vi "Amplifier.vi"(8 "error in (no error)":errorcluster, 10 "Waveform in":waveform(dbl), 11 "RFID system in":refnum<class "RFID system.lvclass">) -> (0 "error out":errorcluster, 2 "Waveform out":waveform(dbl), 3 "RFID system out":refnum<class "RFID system.lvclass">)   [LabVIEW 2019, in "RFID system.lvclass"]
uses:
  RFID system.lvclass
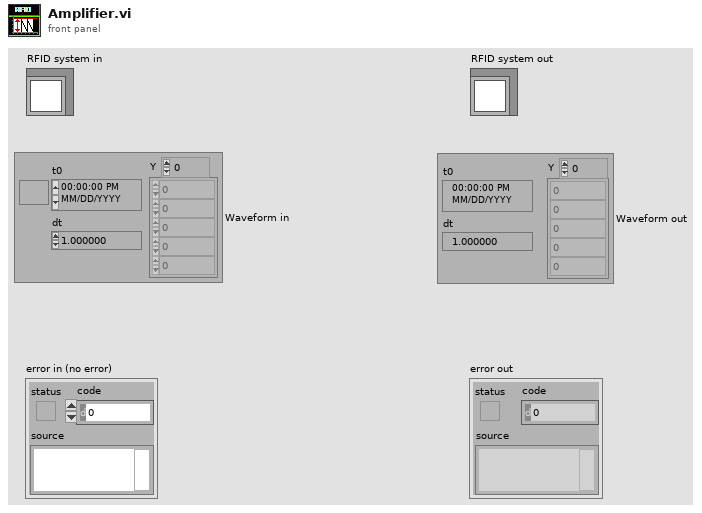
[diagram p1: front panel]
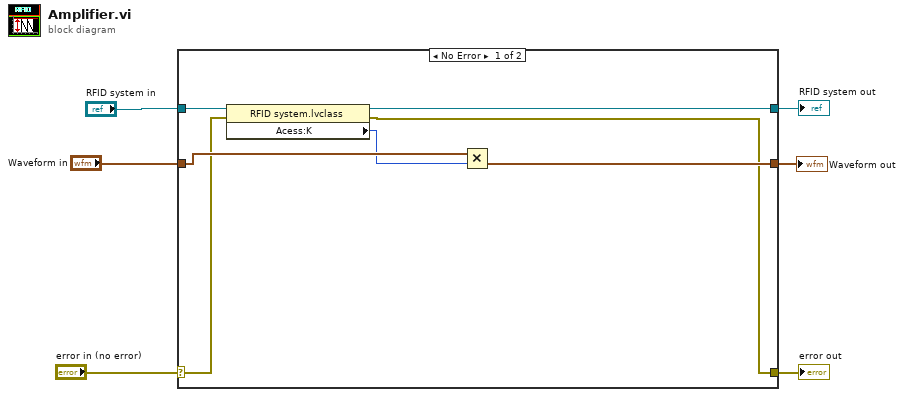
[diagram p0: block diagram]
diagram:
  n1 = case shown="No Error" "error in (no error)" {
    selector: "error in (no error)" -> [w8 w16]
    tunnel: [w7 w16] -> w5
    tunnel: [w9 w15] -> w3
    tunnel: "RFID system in" -> [w13 w15]
    tunnel: "Waveform in" -> [w11 w14]
    tunnel: [w12 w14] -> w1
    frame No Error {
      n2 = property class="RFID system.lvclass"(reference=w13, error in=w8) -> (reference out=w9:refnum<class "RFID system.lvclass">, error out=w7:errorcluster, "Acess:K"=w10:i64)
      n3 = Multiply(x=w11, y=w10) -> (x*y=w12:waveform(dbl))
    }
    frame Error {
    }
  }
  "error out" <- w5
  "RFID system out" <- w3
  "Waveform out" <- w1
